vi "Cleanup.vi"(8 "error in (no error)":errorcluster, 11 "Flex UI (Actor) in":refnum<class "Flex UI (Actor).lvclass">) -> (0 "error out":errorcluster, 3 "Flex UI (Actor) out":refnum<class "Flex UI (Actor).lvclass">)   [LabVIEW 2016, in "Flex UI (Parent Actor).lvlib" / "Flex UI (Actor).lvclass"]
uses:
  Flex UI (Actor).lvclass
  <vilib>/East West Architects/Flex UI/Flex UI (Parent)/Flex UI.lvclass
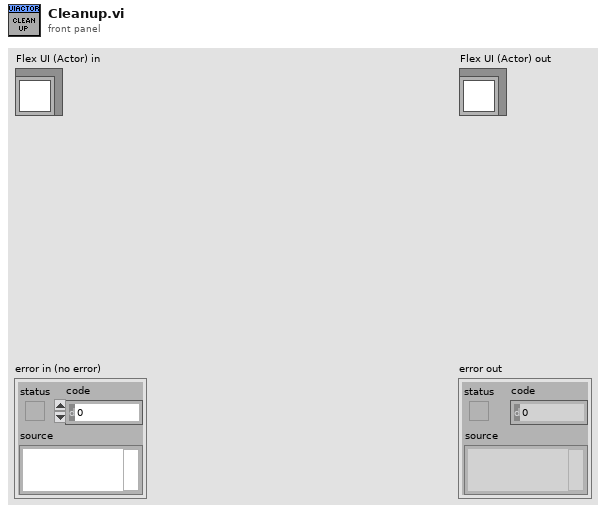
[diagram p1: front panel]
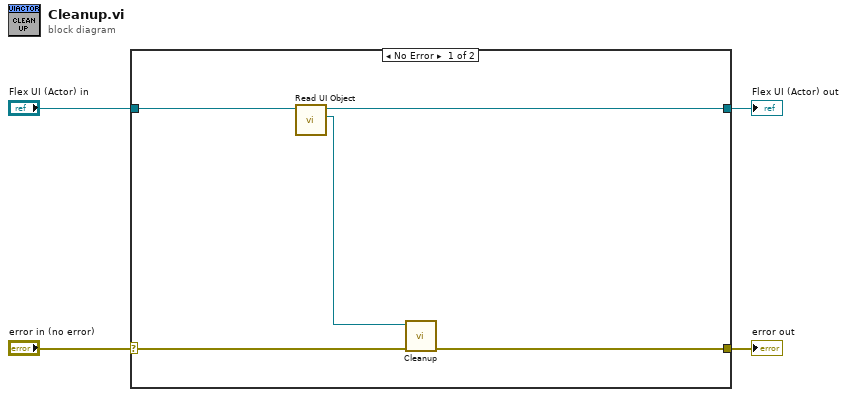
[diagram p0: block diagram]
diagram:
  n1 = case shown="No Error" "error in (no error)" {
    selector: "error in (no error)" -> [w9 w11]
    tunnel: [w5 w11] -> w3
    tunnel: [w6 w10] -> w1
    tunnel: "Flex UI (Actor) in" -> [w8 w10]
    frame No Error {
      n2 = call-dynamic "Read UI Object.vi"("Flex UI (Actor) in"=w8) -> ("Flex UI Object"=w7:refnum<class "Flex UI.lvclass">, "Flex UI (Actor) out"=w6:refnum<class "Flex UI (Actor).lvclass">)  [unwired: 8 in, 1 out]
      n3 = call-dynamic "Cleanup.vi"("error in"=w9, "Flex UI in"=w7) -> ("error out"=w5:errorcluster)  [unwired: 9 in]
    }
    frame Error {
    }
  }
  "error out" <- w3
  "Flex UI (Actor) out" <- w1
